vi "Min Image (SubVI).vi"(8 "Min Image In":u8[](array[numeric]), 9 "Data to Disk":T1, 11 "First Frame?":bool) -> (0 "Min Image":u8[](array[numeric]))   [LabVIEW 2015]
uses:
  Controls (HOST)/Data to Disk Bundle.ctl
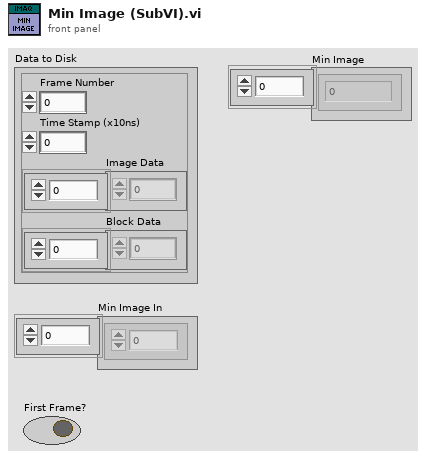
[diagram p1: front panel]
types:
  T1 = typedef "Data to Disk Bundle.ctl" = cluster{"Frame Number":u64, "Time Stamp (x10ns)":u64, "Image Data":u64[], "Block Data":u64[]}
  T2 = enum16{"big-endian, network order", "native, host order", "little-endian"}
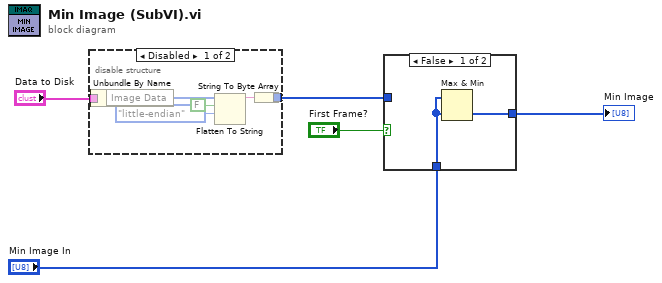
[diagram p0: block diagram]
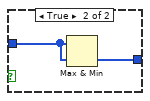
[diagram p3: hidden frame]
diagram:
  n1 = disable-structure shown="Disabled" {
    disable-tunnel: "Data to Disk" -> [w11 _]
    disable-tunnel: [w6 _] -> w3
    frame Disabled {
      n2 = Unbundle By Name(w11) -> ("Image Data"=w10:u64[])
      n3 = Flatten To String(anything=w10, prepend array or string size? (T)=FALSE, byte order (0:big-endian, network order)=T2."little-endian") -> (data string=w7:string)  [unwired: 1 in, 2 out]
      n4 = String To Byte Array(string=w7) -> (unsigned byte array=w6:u8[])
    }
    frame Enabled {
    }
  }
  n5 = case shown="False" "First Frame?" {
    tunnel: "Min Image In" -> [w12 _]
    tunnel: [w13 w15] -> w1
    tunnel: w3 -> [_ w14]
    frame False {
      n6 = Max & Min(x=w12, y=w12) -> (min(x,y)=w13:u8[])  [unwired: 1 out]
    }
    frame True {
      n7 = Max & Min(x=w14, y=w14) -> (min(x,y)=w15:u8[])  [unwired: 1 out]
    }
  }
  "Min Image" <- w1
